vi "UDP_receive_001.vi"() -> ()   [LabVIEW 2019]
panel:
  out "value":dbl
  out "data out":string
  in  "stop":bool
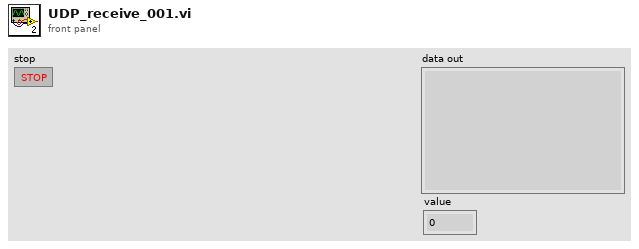
[diagram p1: front panel]
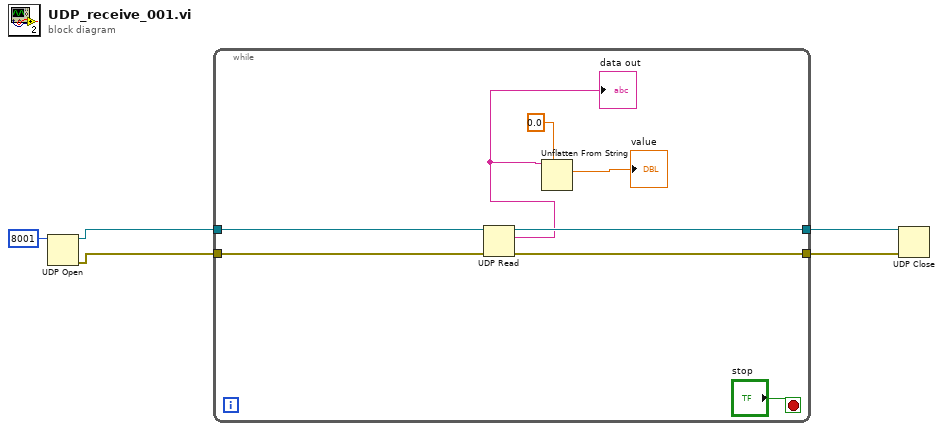
[diagram p0: block diagram]
diagram:
  n1 = UDP Open(11:u16 8001 ("port")) -> (port=w5:refnum<k16>, 0:w3:errorcluster)  [unwired: 4 in, 1 out]
  n2 = while {
    tunnel: w5 -> [w12]
    tunnel: [w11] -> w4
    tunnel: w3 -> [w10]
    tunnel: [w9] -> w2
    stop <- "stop" stop-if-true
    n3 = UDP Read(connection ID=w12, 8:w10) -> (data out=w6:string, error out=w9:errorcluster, 3:w11:refnum<k16>)  [unwired: 2 in, 2 out]
    "data out" <- w6
    n4 = Unflatten From String(type=0.0, binary string=w6) -> (value=→"value":dbl)  [unwired: 3 in, 2 out]
  }
  n5 = UDP Close(connection ID=w4, 8:w2) -> ()  [unwired: 2 out]
